vi "GetName.vi"(8 "error in (no error)":errorcluster, 11 "reference in":refnum<class "TAFBaseGUI.lvclass">) -> (0 "error out":errorcluster, 2 "Name":string, 3 "reference out":refnum<class "TAFBaseGUI.lvclass">)   [LabVIEW 2021, in "TAFBaseGUI.lvclass"]
uses:
  TAFBaseGUI.lvclass
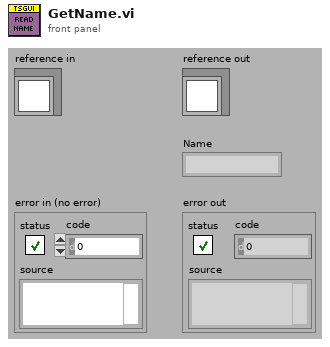
[diagram p1: front panel]
types:
  T1 = typedef "TAFBaseGUI.lvclass/ObjectAttributes.ctl" = cluster{"Name":string, "FPVIRef":refnum<vi>}
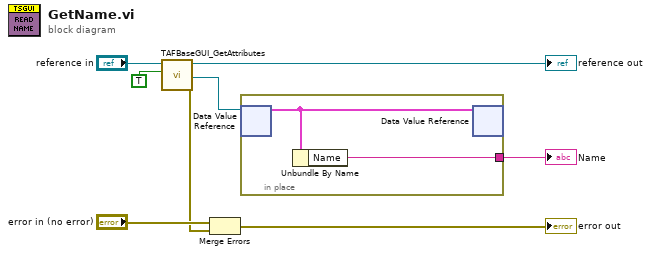
[diagram p0: block diagram]
diagram:
  n1 = call "TAFBaseGUI_GetAttributes.vi"("OnlyGetDvrReference(False)"=TRUE, "reference in"="reference in") -> ("error out"=w5:errorcluster, "DataRef"=w2:refnum<data-value>, "reference out"=→"reference out":refnum<class "TAFBaseGUI.lvclass">)  [unwired: 6 in, 1 out]
  n2 = Merge Errors("error in (no error)", w5) -> (→"error out":errorcluster)
  n3 = in-place {
    in-place-border: [w10] -> w1
    n4 = in-place-dvr #1(w2) -> (w9:T1)  [unwired: 1 out]
    n5 = Unbundle By Name(w9) -> ("Name"=w10:string)
    n6 = in-place-dvr #1(w9) -> ()  [unwired: 2 out]
  }
  "Name" <- w1
